vi "Rectangel MoveRectToFreeSpace.vi"(1 "BoundsArray":T3[](array[typedef]) {"height" format="%.2f"; "width" format="%.2f"; "y" format="%.2f"; "x" format="%.2f"}, 2 "bounds":T3 {"height" format="%.2f"; "width" format="%.2f"; "y" format="%.2f"; "x" format="%.2f"}, 5 "error in (no error)":errorcluster, 8 "DirectionsToTest(E-S-W-N)":T1) -> (15 "Found":bool, 16 "BoundsOut":T3 {"height" format="%.2f"; "width" format="%.2f"; "y" format="%.2f"; "x" format="%.2f"}, 17 "point":T2 {"y" format="%.2f"; "x" format="%.2f"}, 19 "error out":errorcluster)   [LabVIEW 2020]
doc: "contains"
uses:
  <resource>/Framework/Providers/Open_GDS/UML/General/Rectangle/Rectangle Rectangle2D.ctl
  <resource>/Framework/Providers/Open_GDS/UML/General/Point/Point Point2D.ctl
  <resource>/Framework/Providers/Open_GDS/UML/General/Rectangle/Rectangle DirectionToTest.ctl
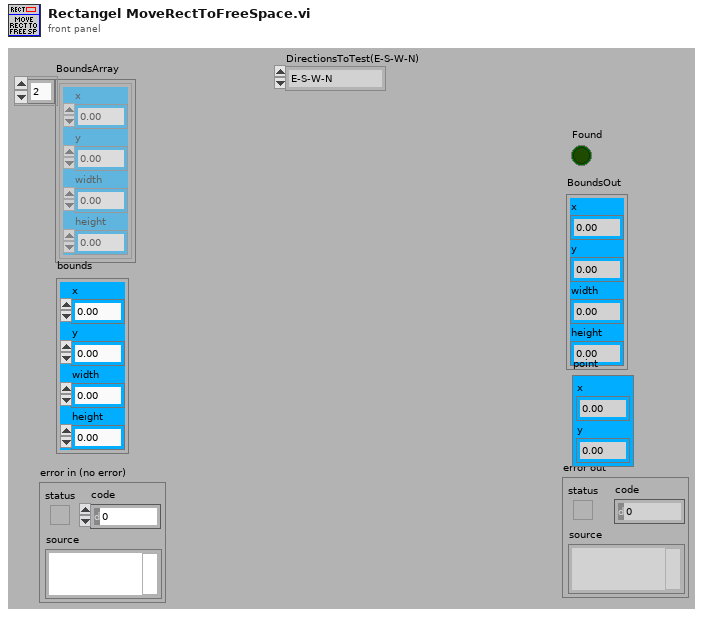
[diagram p1: front panel]
types:
  T1 = typedef "Rectangle DirectionToTest.ctl" = enum16{"E-S-W-N", "ES-S-WS"}
  T2 = typedef "Point Point2D.ctl" = cluster{"x":dbl, "y":dbl}
  T3 = typedef "Rectangle Rectangle2D.ctl" = cluster{"x":dbl, "y":dbl, "width":dbl, "height":dbl}
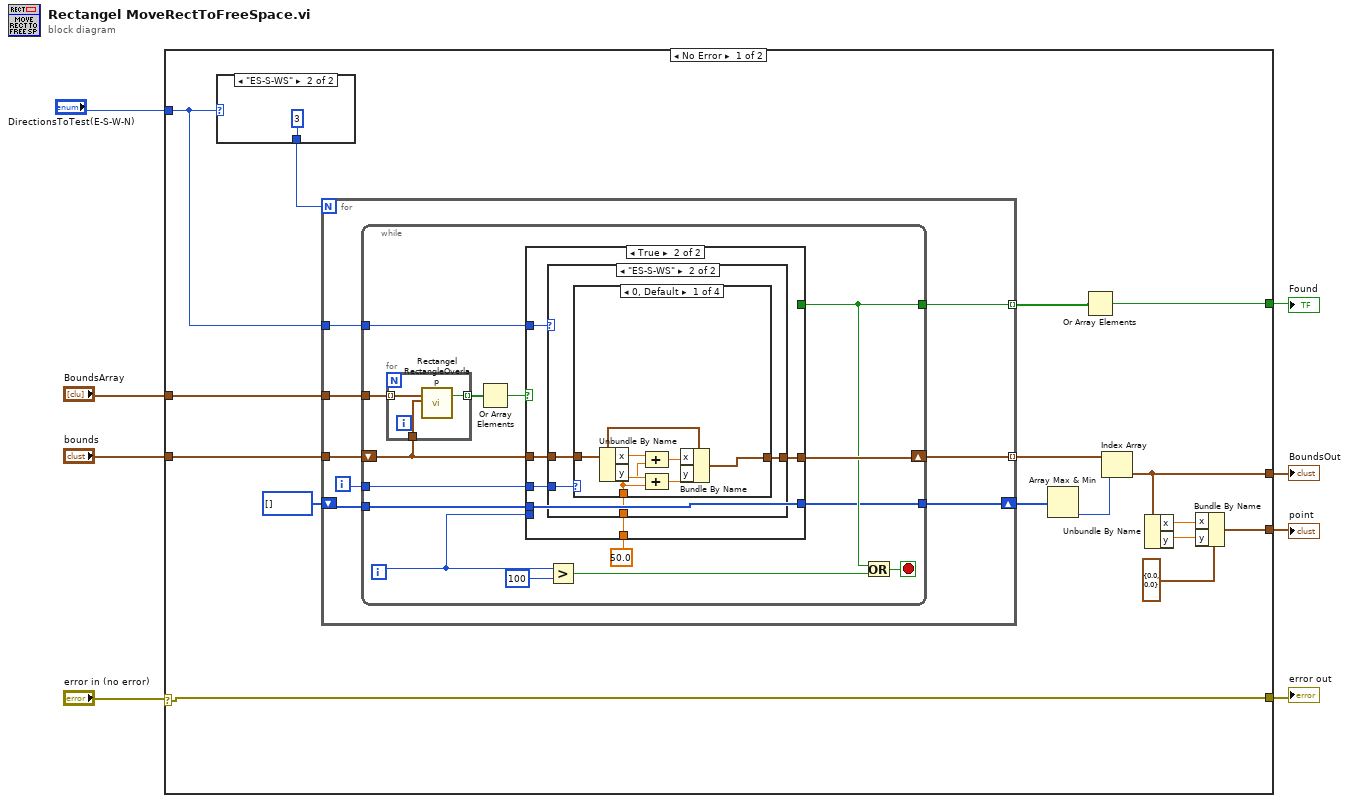
[diagram p0: block diagram]
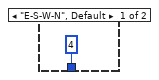
[diagram p2: hidden frame]
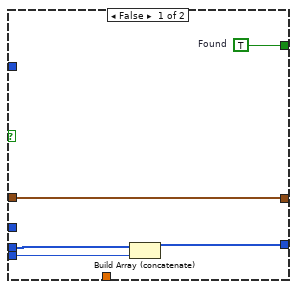
[diagram p3: hidden frame]
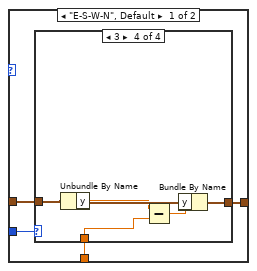
[diagram p4: hidden frame]
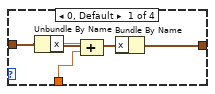
[diagram p5: hidden frame]
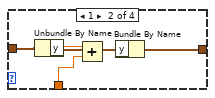
[diagram p6: hidden frame]
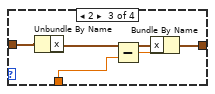
[diagram p7: hidden frame]
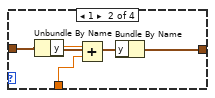
[diagram p8: hidden frame]
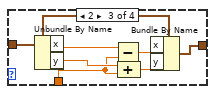
[diagram p9: hidden frame]
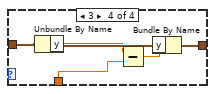
[diagram p10: hidden frame]
diagram:
  n1 = case shown="No Error" "error in (no error)" {
    selector: "error in (no error)" -> [w11 w116]
    tunnel: [w11 w116] -> w8
    tunnel: "BoundsArray" -> [w24 _]
    tunnel: "bounds" -> [w21 _]
    tunnel: [w22 _] -> w4
    tunnel: [w16 _] -> w3
    tunnel: [w13 _] -> w2
    tunnel: "DirectionsToTest(E-S-W-N)" -> [w9 _]
    frame No Error {
      n2 = case shown="\"ES-S-WS\"" w9 {
        tunnel: [4 3] -> w10
        frame "E-S-W-N", Default {
        }
        frame "ES-S-WS" {
        }
      }
      n3 = for {
        N: w10 -> [_]
        tunnel: w24 -> [w34]
        tunnel: w21 -> [w33]
        tunnel: [w31] -> w23 mode=indexing
        tunnel: [w30] -> w19 mode=indexing
        shift-right: [w28] -> w20
        shift-left: i32[] [] -> [w29]
        tunnel: w9 -> [w27]
        i -> [w32]
        n4 = while {
          tunnel: w34 -> [w39]
          shift-right: [w48] -> w30
          shift-left: w33 -> [w40]
          tunnel: w32 -> [w49]
          tunnel: [w44] -> w31
          tunnel: w29 -> [w43]
          tunnel: [w41] -> w28
          tunnel: w27 -> [w35]
          i -> [w42]
          stop <- w45 stop-if-true
          n5 = for {
            tunnel: [w52] -> w38 mode=indexing
            tunnel: w40 -> [w51]
            tunnel: w39 -> [w50] mode=indexing
            n6 = call <resource>:"Rectangel RectangleOverlap.vi"("bounds1"=w50, "bounds2"=w51) -> ("overlap"=w52:bool)  [unwired: 2 in, 15 out]
          }
          n7 = Or Array Elements(Boolean array=w38) -> (logical OR=w37:bool)
          n8 = case shown="True" w37 {
            tunnel: w49 -> [_ w63]
            tunnel: w40 -> [w57 w62]
            tunnel: [w57 w61] -> w48
            tunnel: [w56 _] -> w44
            tunnel: w43 -> [w55 w60]
            tunnel: w42 -> [w54 _]
            tunnel: [w53 w60] -> w41
            tunnel: 50.0 ("y") -> [_ w59]
            tunnel: w35 -> [_ w58]
            frame False {
              w56 = TRUE  # Found
              n9 = Build Array (concatenate)(w55, w54) -> (w53:i32[])
            }
            frame True {
              n10 = case shown="\"ES-S-WS\"" w58 {
                tunnel: w63 -> [w67 w91]
                tunnel: w62 -> [w66 w90]
                tunnel: [w65 w89] -> w61
                tunnel: w59 -> [w64 w88]
                frame "E-S-W-N", Default {
                  n11 = case shown="3" w67 {
                    tunnel: w66 -> [w72 w77 w82 w87]
                    tunnel: [w70 w75 w81 w86] -> w65
                    tunnel: w64 -> [w68 w73 w78 w83]
                    frame 0, Default {
                      n12 = Unbundle By Name(w72) -> ("x"=w69:dbl)
                      n13 = Compound Arithmetic op=ADD(w69, w68) -> (w71:dbl)
                      n14 = Bundle By Name(cluster=w72, "x"=w71) -> (w70:T3)
                    }
                    frame 1 {
                      n15 = Unbundle By Name(w77) -> ("y"=w74:dbl)
                      n16 = Add(x=w74, y=w73) -> (x+y=w76:dbl)
                      n17 = Bundle By Name(cluster=w77, "y"=w76) -> (w75:T3)
                    }
                    frame 2 {
                      n18 = Unbundle By Name(w82) -> ("x"=w79:dbl)
                      n19 = Subtract(x=w79, y=w78) -> (x-y=w80:dbl)
                      n20 = Bundle By Name(cluster=w82, "x"=w80) -> (w81:T3)
                    }
                    frame 3 {
                      n21 = Unbundle By Name(w87) -> ("y"=w84:dbl)
                      n22 = Subtract(x=w84, y=w83) -> (x-y=w85:dbl)
                      n23 = Bundle By Name(cluster=w87, "y"=w85) -> (w86:T3)
                    }
                  }
                }
                frame "ES-S-WS" {
                  n24 = case shown="0, Default" w91 {
                    tunnel: w90 -> [w98 w103 w110 w115]
                    tunnel: [w97 w101 w109 w114] -> w89
                    tunnel: w88 -> [w93 w99 w105 w111]
                    frame 0, Default {
                      n25 = Unbundle By Name(w98) -> ("x"=w96:dbl, "y"=w94:dbl)
                      n26 = Compound Arithmetic op=ADD(w96, w93) -> (w95:dbl)
                      n27 = Compound Arithmetic op=ADD(w94, w93) -> (w92:dbl)
                      n28 = Bundle By Name(cluster=w98, "x"=w95, "y"=w92) -> (w97:T3)
                    }
                    frame 1 {
                      n29 = Unbundle By Name(w103) -> ("y"=w100:dbl)
                      n30 = Add(x=w100, y=w99) -> (x+y=w102:dbl)
                      n31 = Bundle By Name(cluster=w103, "y"=w102) -> (w101:T3)
                    }
                    frame 2 {
                      n32 = Unbundle By Name(w110) -> ("x"=w107:dbl, "y"=w106:dbl)
                      n33 = Subtract(x=w107, y=w105) -> (x-y=w108:dbl)
                      n34 = Compound Arithmetic op=ADD(w106, w105) -> (w104:dbl)
                      n35 = Bundle By Name(cluster=w110, "x"=w108, "y"=w104) -> (w109:T3)
                    }
                    frame 3 {
                      n36 = Unbundle By Name(w115) -> ("y"=w112:dbl)
                      n37 = Subtract(x=w112, y=w111) -> (x-y=w113:dbl)
                      n38 = Bundle By Name(cluster=w115, "y"=w113) -> (w114:T3)
                    }
                  }
                }
              }
            }
          }
          n39 = Greater?(x=w42, y=100) -> (0:w46:bool)
          n40 = Or(x=w44, y=w46) -> (x .or. y?=w45:bool)
        }
      }
      n41 = Array Max & Min(array=w20) -> (min index (indices)=w18:i32)  [unwired: 3 out]
      n42 = Or Array Elements(Boolean array=w23) -> (logical OR=w22:bool)
      n43 = Index Array(array=w19, index=w18) -> (element=w16:T3)
      n44 = Unbundle By Name(w16) -> ("x"=w15:dbl, "y"=w14:dbl)
      n45 = Bundle By Name(cluster=T2 {"x"=0.0, "y"=0.0} ("point"), "x"=w15, "y"=w14) -> (w13:T2)
    }
    frame Error {
    }
  }
  "error out" <- w8
  "Found" <- w4
  "BoundsOut" <- w3
  "point" <- w2
